vi "Camera startup.vi"() -> ()   [LabVIEW 2016]
doc: "Cools down the camera to operating temperature before use and returns it to ambient after use. Run this VI before running any other ixon programs and leave it running the whole time you use the camera. To start: run vi, set temperature, check \"cooling\". To finish: Click \"warm up CCD and turn off camera\". Leave running until the program tells you that it has turned off the camera."
uses:
  ixon camera/HAL camera properties.ctl
  ixon camera/HAL cooling status.ctt
  ixon ultra 897/HAL Camera specifications globals.vi
  camera globals.vi
panel:
  out "Cooling status":T1
  in  "Warm up CCD & Turn Off Camera":bool
  in  "Cooling":bool
  out "Detector Temperature":i32(graph)
  in  "Temp. Set Point":i32(slide)=-70 scale=-120.0..20.0
  out "Camera Properties":T2
  out "Status":string
  in  "error in (no error)":errorcluster
  # "Camera:  Andor iXon/iXon Ultra"
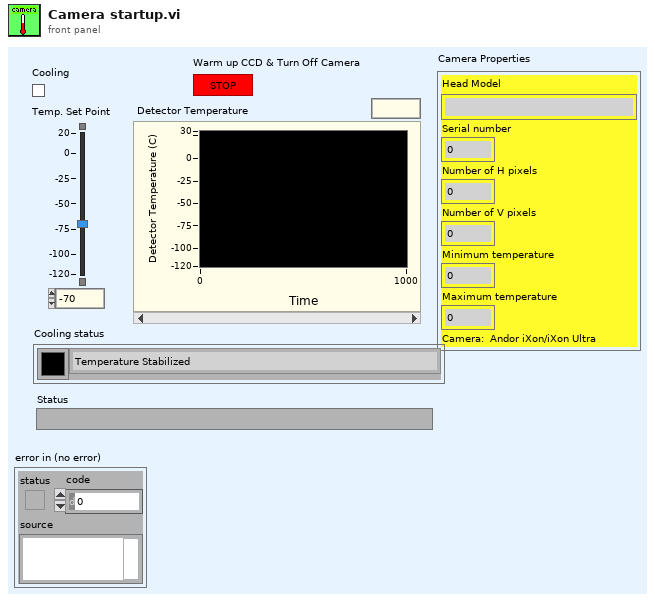
[diagram p1: front panel]
types:
  T1 = typedef "HAL cooling status.ctt" = cluster{"Color Box":u32, "Cooling Status":enum16{"Temperature Stabilized", "Waiting to Stabilize Temperature", "Cooling is Turned Off", "Have not yet Reached Set Temperature"}}
  T2 = typedef "HAL camera properties.ctl" = cluster{"Head Model":string, "Serial number":i32, "Number of H pixels":i32, "Number of V pixels":i32, "Minimum temperature":i32, "Maximum temperature":i32}
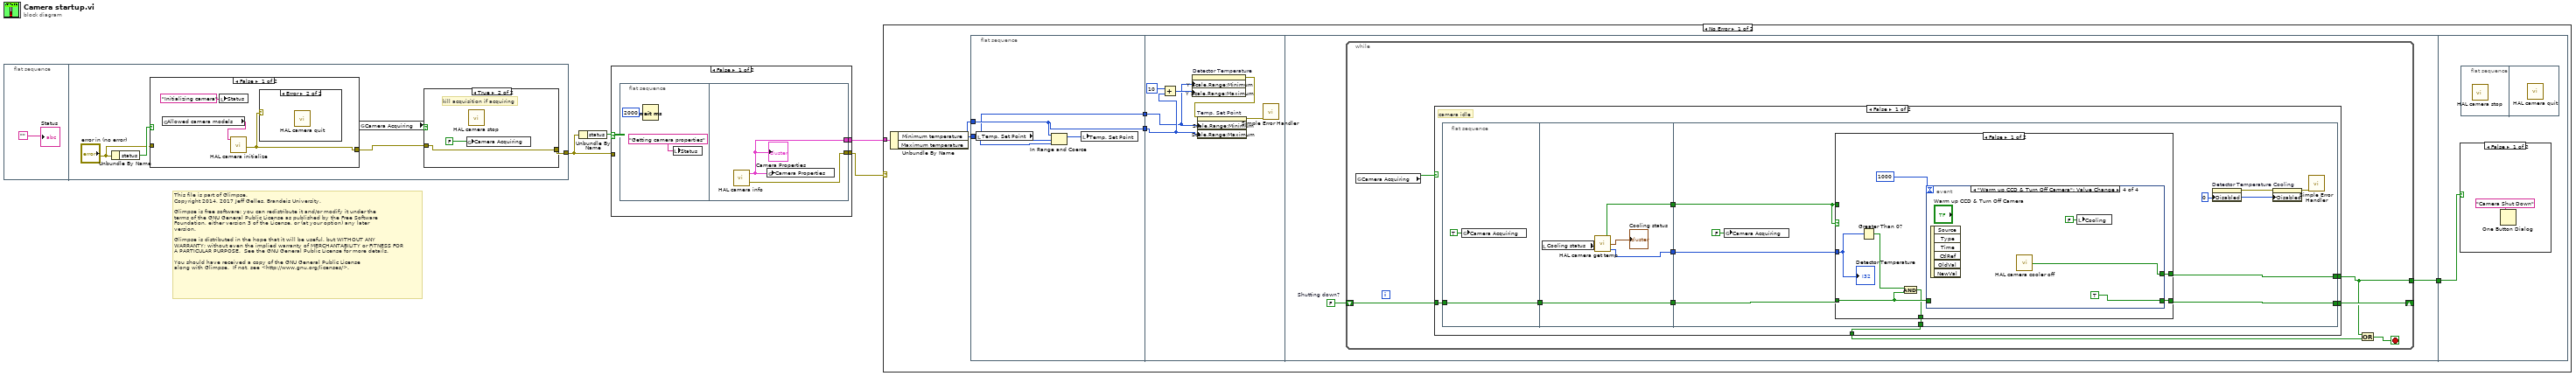
[diagram p0: block diagram]
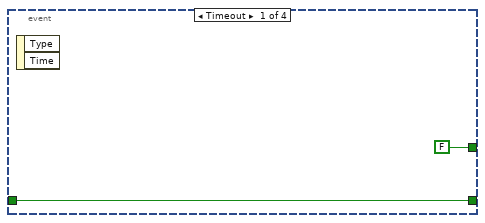
[diagram p5: hidden frame]
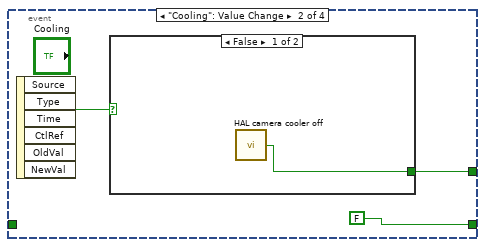
[diagram p6: hidden frame]
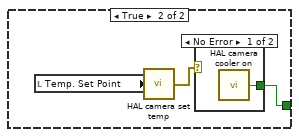
[diagram p7: hidden frame]
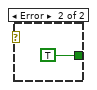
[diagram p8: hidden frame]
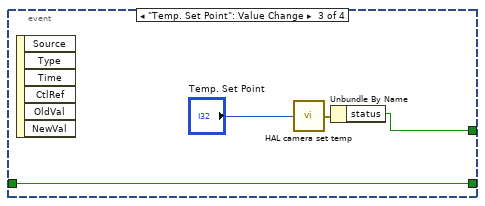
[diagram p9: hidden frame]
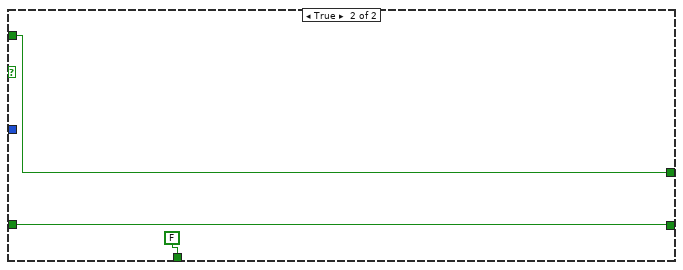
[diagram p10: hidden frame]
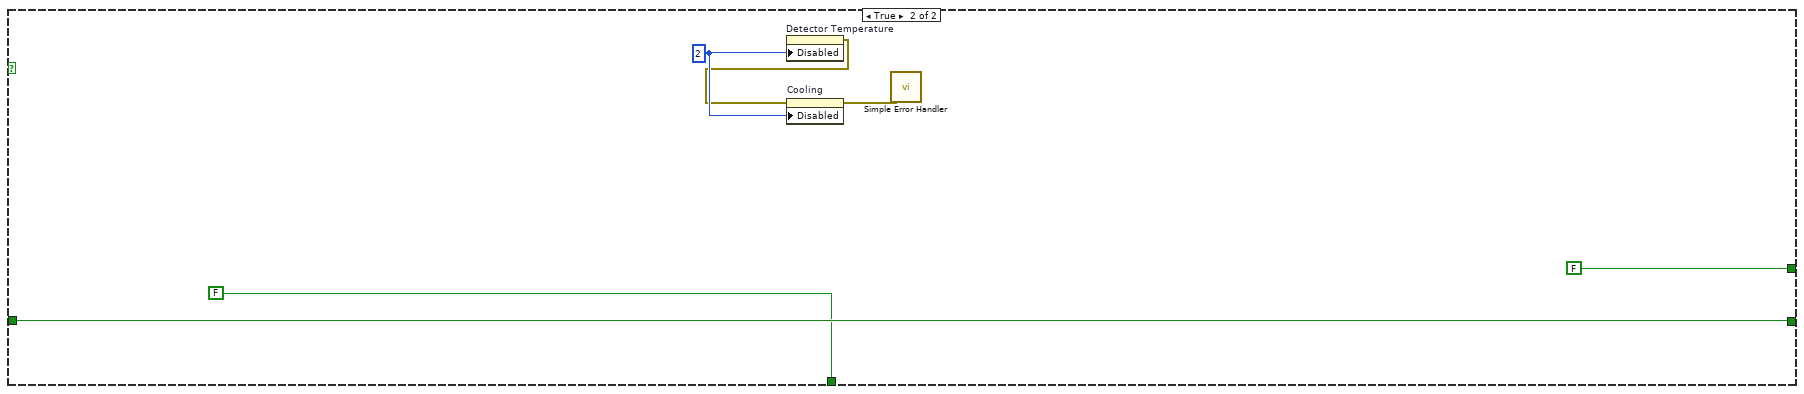
[diagram p11: hidden frame]
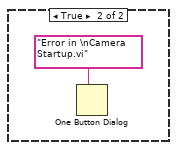
[diagram p12: hidden frame]
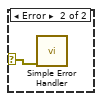
[diagram p13: hidden frame]
diagram:
  # "This file is part of Glimpse. \nCopyright 2014, 2017 Jeff Gelles, Brandeis University.    \n\nGlimpse is free software: you can redistribute it and/or modify it under the \nterms of the GNU General Public License as published by the Free Software \nFoundation, either version 3 of the License, or (at your option) any later \nversion.\n\nGlimpse is distributed in the hope that it will be useful, but WITHOUT ANY \nWARRANTY; without even the implied warranty of MERCHANTABILITY or FITNESS FOR \nA PARTICULAR PURPOSE.  See the GNU General Public License for more details.\n\nYou should have received a copy of the GNU General Public License\nalong with Glimpse.  If not, see <http://www.gnu.org/licenses/>."
  n1 = flat-sequence {
    tunnel: [w7] -> w3
    frame #0 {
      "Status" <- ""
    }
    frame #1 {
      n2 = Unbundle By Name("error in (no error)") -> ("status"=w10:bool)
      n3 = case shown="False" w10 {
        tunnel: [w15 w17] -> w8
        tunnel: "error in (no error)" -> [_ w17]
        frame False {
          n4 = global read "HAL Camera specifications globals.vi" "Allowed camera models"() -> (w14:string[])
          n5 = local write "Status"("Initializing camera" ("Status")) -> ()
          n6 = call "HAL camera initialize.vi"("Select camera model(s)"=w14) -> ("error out"=w15:errorcluster)  [unwired: 6 in]
          n7 = case shown="Error" w15 {
            frame No Error {
            }
            frame Error {
              n8 = call "HAL camera quit.vi"() -> ()  [unwired: 1 out]
            }
          }
        }
        frame True {
        }
      }
      n9 = global read "camera globals.vi" "Camera Acquiring"() -> (w6:bool)
      n10 = case shown="True" w6 {
        tunnel: [w11 w13] -> w7
        tunnel: w8 -> [w11 w13]
        frame False {
        }
        frame True {
          # "kill acquisition if acquiring"
          n11 = global write "camera globals.vi" "Camera Acquiring"(FALSE ("Andor Aquiring")) -> ()
          n12 = call "HAL camera stop.vi"() -> ()  [unwired: 1 out]
        }
      }
    }
  }
  n13 = Unbundle By Name(w3) -> ("status"=w4:bool)
  n14 = case shown="False" w4 {
    tunnel: [w18 w24] -> w1
    tunnel: w3 -> [_ w24]
    tunnel: [w19 _] -> w2
    frame False {
      n15 = flat-sequence {
        tunnel: [w22] -> w19
        tunnel: [w23] -> w18
        frame #0 {
          n16 = Wait (ms)(milliseconds to wait=u32 2000) -> ()  [unwired: 1 out]
          n17 = local write "Status"("Getting camera properties" ("Status")) -> ()
        }
        frame #1 {
          n18 = call "HAL camera info.vi"() -> ("error out"=w23:errorcluster, "Andor Camera Properties"=w22:T2)  [unwired: 2 in]
          "Camera Properties" <- w22
          n19 = global write "camera globals.vi" "Camera Properties"(w22) -> ()
        }
      }
    }
    frame True {
    }
  }
  n20 = case shown="No Error" w1 {
    selector: w1 -> [_ w111]
    tunnel: w2 -> [w30 _]
    frame No Error {
      n21 = Unbundle By Name(w30) -> ("Minimum temperature"=w26:i32, "Maximum temperature"=w28:i32)
      n22 = flat-sequence {
        tunnel: w28 -> [w32]
        tunnel: [w32] -> w27
        tunnel: w26 -> [w31]
        tunnel: [w31] -> w25
        tunnel: w27 -> [w36]
        tunnel: w25 -> [w35]
        tunnel: [w41] -> w29
        tunnel: w29 -> [w108]
        frame #0 {
          n23 = local read "Temp. Set Point"() -> (w34:i32)
          n24 = In Range and Coerce(upper limit=w32, x=w34, lower limit=w31) -> (coerced(x)=w33:i32)  [unwired: 1 out]
          n25 = local write "Temp. Set Point"(w33) -> ()
        }
        frame #1 {
          n26 = Add(x=10, y=w36) -> (x+y=w39:i32)
          n27 = property on="Detector Temperature" class="WFChart (strict)"("Y Scale.Range:Minimum"=w35, "Y Scale.Range:Maximum"=w39) -> (error out=w38:errorcluster)  [unwired: 2 in, 1 out]
          n28 = property on="Temp. Set Point" class="Slide (strict)"(error in=w38, "Scale.Range:Minimum"=w35, "Scale.Range:Maximum"=w36) -> (error out=w37:errorcluster)  [unwired: 1 in, 1 out]
          n29 = call <vilib>:"Simple Error Handler.vi"("error in (no error)"=w37) -> ()  [unwired: 1 in, 8 out]
        }
        frame #2 {
          w42 = FALSE  # Shutting down?
          n30 = while {
            shift-right: [w46] -> _
            shift-left: w42 -> [w47]
            tunnel: [w43] -> w41
            stop <- w44 stop-if-true
            n31 = global read "camera globals.vi" "Camera Acquiring"() -> (w48:bool)
            n32 = case shown="False" w48 {
              tunnel: w47 -> [w53 w105]
              tunnel: [w56 w105] -> w46
              tunnel: [w55 FALSE] -> w45
              tunnel: [w54 FALSE ("status")] -> w43
              frame False {
                # "camera idle"
                n33 = flat-sequence {
                  tunnel: w53 -> [w58]
                  tunnel: [w58] -> w52
                  tunnel: w52 -> [w63]
                  tunnel: [w63] -> w51
                  tunnel: [w60] -> w50
                  tunnel: [w59] -> w49
                  tunnel: [w70] -> w56
                  tunnel: [w69] -> w55
                  tunnel: [w68] -> w54
                  tunnel: w51 -> [w67]
                  tunnel: w50 -> [w66]
                  tunnel: w49 -> [w65]
                  frame #0 {
                    n34 = global write "camera globals.vi" "Camera Acquiring"(TRUE ("Camera Acquiring")) -> ()
                  }
                  frame #1 {
                    n35 = local read "Cooling status"() -> (w62:T1)
                    n36 = call "HAL camera get temp.vi"("Cooling status In"=w62) -> ("Error?"=w60:bool, "Cooling status Out"=→"Cooling status":T1, "Current temperature"=w59:i32)
                  }
                  frame #2 {
                    w73 = u8 0 ("Disabled")
                    n37 = global write "camera globals.vi" "Camera Acquiring"(FALSE ("Camera Acquiring")) -> ()
                    n38 = case shown="False" w66 {
                      tunnel: [w79 w99] -> w70
                      tunnel: w67 -> [w78 w99]
                      tunnel: w65 -> [w77 _]
                      tunnel: [w75 FALSE] -> w69
                      tunnel: [w74 w101] -> w68
                      tunnel: w66 -> [_ w101]
                      frame False {
                        n39 = Greater Than 0?(x=w77) -> (x > 0?=w76:bool)
                        n40 = And(x=w76, y=w78) -> (x .and. y?=w75:bool)
                        n41 = event shown="[3] \"Warm up CCD & Turn Off Camera\": Value Change" {
                          selector: _ -> [_ _ _ _]
                          dyn-events: _ -> [_ _ _ _]
                          timeout: 1000 -> [_ _ _ _]
                          tunnel: w78 -> [w82 _ w92 _]
                          tunnel: [w82 FALSE w92 TRUE] -> w79
                          tunnel: [FALSE ("status") w84 w93 w97] -> w74
                          event Timeout {
                            n42 = event-data() -> ()  [unwired: 3 out]
                          }
                          event "Cooling": Value Change {
                            n43 = event-data() -> ("NewVal"=w83:bool)  [unwired: 6 out]
                            n44 = case shown="False" w83 {
                              tunnel: [w86 w89] -> w84
                              frame False {
                                n45 = call "HAL camera cooler off.vi"() -> ("Error?"=w86:bool)
                              }
                              frame True {
                                n46 = local read "Temp. Set Point"() -> (w88:i32)
                                n47 = call "HAL camera set temp.vi"("Temp. Set Point"=w88) -> ("error out"=w87:errorcluster)
                                n48 = case shown="No Error" w87 {
                                tunnel: [w90 TRUE ("error?")] -> w89
                                frame No Error {
                                n49 = call "HAL camera cooler on.vi"() -> ("error?"=w90:bool)
                                }
                                frame Error {
                                }
                                }
                              }
                            }
                          }
                          event "Temp. Set Point": Value Change {
                            n50 = event-data() -> ()  [unwired: 7 out]
                            n51 = call "HAL camera set temp.vi"("Temp. Set Point"="Temp. Set Point") -> ("error out"=w94:errorcluster)
                            n52 = Unbundle By Name(w94) -> ("status"=w93:bool)
                          }
                          event "Warm up CCD & Turn Off Camera": Value Change {
                            n53 = event-data() -> ()  [unwired: 7 out]
                            n54 = call "HAL camera cooler off.vi"() -> ("Error?"=w97:bool)
                            n55 = local write "Cooling"(FALSE ("Cooling")) -> ()
                          }
                        }
                        "Detector Temperature" <- w77
                      }
                      frame True {
                      }
                    }
                    n56 = property on="Detector Temperature" class="WFChart (strict)"("Disabled"=w73) -> (error out=w72:errorcluster)  [unwired: 2 in, 1 out]
                    n57 = property on="Cooling" class="Bool (strict)"(error in=w72, "Disabled"=w73) -> (error out=w71:errorcluster)  [unwired: 1 in, 1 out]
                    n58 = call <vilib>:"Simple Error Handler.vi"("error in (no error)"=w71) -> ()  [unwired: 1 in, 8 out]
                  }
                }
              }
              frame True {
                w107 = u8 2 ("Disabled")
                n59 = property on="Detector Temperature" class="WFChart (strict)"("Disabled"=w107) -> (error out=w106:errorcluster)  [unwired: 2 in, 1 out]
                n60 = property on="Cooling" class="Bool (strict)"(error in=w106, "Disabled"=w107) -> (error out=w102:errorcluster)  [unwired: 1 in, 1 out]
                n61 = call <vilib>:"Simple Error Handler.vi"("error in (no error)"=w102) -> ()  [unwired: 1 in, 8 out]
              }
            }
            n62 = Compound Arithmetic op=OR(w43, w45) -> (w44:bool)
          }
        }
        frame #3 {
          n63 = case shown="False" w108 {
            frame False {
              n64 = One Button Dialog(message="Camera Shut Down" ("string")) -> ()  [unwired: 2 out]
            }
            frame True {
              n65 = One Button Dialog(message="Error in \nCamera Startup.vi" ("string")) -> ()  [unwired: 2 out]
            }
          }
          n66 = flat-sequence {
            frame #0 {
              n67 = call "HAL camera stop.vi"() -> ()  [unwired: 1 in]
            }
            frame #1 {
              n68 = call "HAL camera quit.vi"() -> ()  [unwired: 1 out]
            }
          }
        }
      }
    }
    frame Error {
      n69 = call <vilib>:"Simple Error Handler.vi"("error in (no error)"=w111) -> ()  [unwired: 1 in, 8 out]
    }
  }
